vi "Get Level.vi"(8 "error in":errorcluster, 11 "LogRecord in":refnum<class "LogRecord.lvclass">) -> (0 "error out":errorcluster, 2 "Level":T1, 3 "LogRecord out":refnum<class "LogRecord.lvclass">)   [LabVIEW 2020, in "hse-logger.lvlib" / "LogRecord.lvclass"]
doc: "Returns the level of this LogRecord.\n\n____\nHAMPEL SOFTWARE ENGINEERING v2.0.6 (2021-04-15 11:38)"
uses:
  LogRecord.lvclass
  LogLevel.ctl
  LogRecord.lvclass/LogRecord.ctl
  hse-logger.lvlib
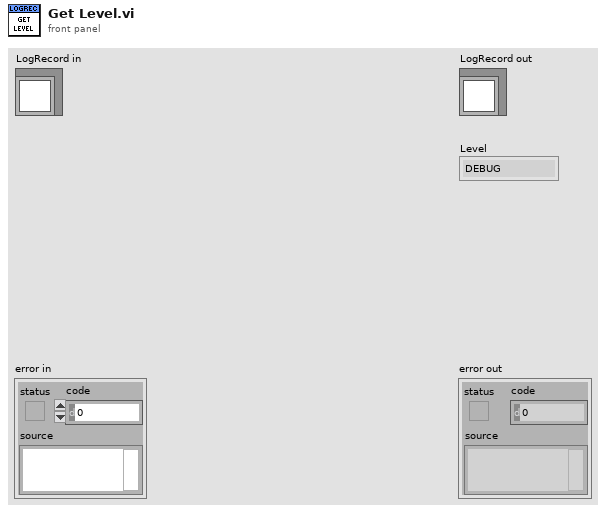
[diagram p1: front panel]
types:
  T1 = typedef "hse-logger.lvlib/LogLevel.ctl" = enum16{"DEBUG", "INFO", "WARNING", "ERROR", "CRITICAL"}
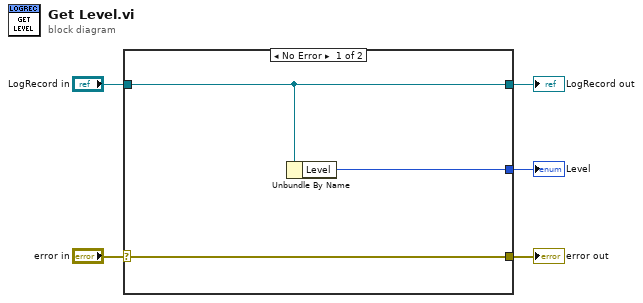
[diagram p0: block diagram]
diagram:
  n1 = case shown="No Error" "error in" {
    selector: "error in" -> [w8 w9]
    tunnel: [w8 w9] -> w4
    tunnel: [w7 w10] -> w2
    tunnel: "LogRecord in" -> [w7 w10]
    tunnel: [w6 _] -> w1
    frame No Error {
      n2 = Unbundle By Name(w7) -> ("Level"=w6:T1)
    }
    frame Error {
    }
  }
  "error out" <- w4
  "LogRecord out" <- w2
  "Level" <- w1
